vi "Import_labview_files.vi"(5 "Convert":bool, 6 "Role ID Array":T3[](array[typedef]), 9 "Hardware ID Array":T2[](array[typedef]), 11 "Folder of Labview files to import:":path=path "\\\\ccldas1.colorado.edu\\Data/Raw_Data/2012_06_16_Lightflash/Labview/run4.1") -> ()   [LabVIEW 2012]
uses:
  Private/Role ID.ctl
  Private/Hardware ID.ctl
  Private/Pelletron.ctl
  Public API/Post_Dust_Event.ctl
  Private/Estimate_source.ctl
  Private/File_location.ctl
  Public API/Signal.ctl
  <vilib>/addons/database/Auxilliary.llb/DB Tools Cursor Type.ctl
  <vilib>/Utility/file.llb/Read From Spreadsheet File (string).vi
  <vilib>/addons/database/Connection.llb/Conn Execute.vi
  <vilib>/addons/database/Recordset.llb/Rec Fetch Recordset Data (R).vi
  <vilib>/addons/database/Recordset.llb/Rec Destroy - Connection.vi
  <vilib>/addons/database/_DB Variant To Data/Database Variant To Data.xnode
  <vilib>/addons/database/NI_Database_API.lvlib
panel:
  in  "Tab Control":T1(tab)
  out "Number of Labview files to be imported:":dbl
  out "Slide":u8(slide) scale=0.0..100.0
  in  "Non-standard termination for 3rd detector?":bool
  in  "Metadata file to import:":path=path "\\\\ccldas1.colorado.edu\\Data/Raw_Data/2012_06_16_Lightflash/Labview/run4.1"
  in  "Convert Metadata":bool
  out "metadata Slide":u8(slide) scale=0.0..100.0
  out "Test":bool caption="Test Database in use:"
  out "Test 2":bool=TRUE caption="Production Database in use:"
  in  "error in (no error)":errorcluster
  out "error out":errorcluster
  in  "stop":bool
  # "CCLDAS Database Import System V2.0"
  # "ODBC Connection Status:"
  # "Error Status:"
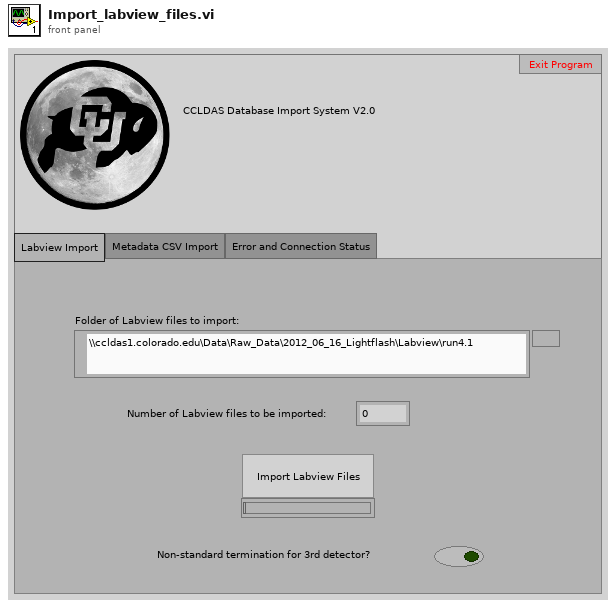
[diagram p1: front panel]
types:
  T1 = enum32{"Labview Import", "Metadata CSV Import", "Error and Connection Status"}
  T2 = typedef "Hardware ID.ctl" = enum16{"Unknown", "CSA 1", "CSA 2", "CSA 3", "CSA 4", "CSA 5", "CSA 6"}
  T3 = typedef "Role ID.ctl" = enum16{"First_Detector", "Second_Detector", "Third_Detector", "LeCroy_CH1", "LeCroy_CH2", "LeCroy_CH3", "LeCroy_CH4", "PSU"}
  T4 = typedef "Post_Dust_Event.ctl" = cluster{"Dust Event ID":i64, "Integer Timestamp":i64, "Velocity":sgl, "Mass":sgl, "Charge":sgl, "Radius":sgl, "Passed_3rd_Detector":i8, "Experiment Settings":dbl, "Pelletron ID":i32, "Estimate Source":T5, "Estimate Quality":sgl, "File Location":T6, "id_dust_info":dbl}
  T5 = typedef "Estimate_source.ctl" = i8
  T6 = typedef "File_location.ctl" = i8
  T7 = typedef "Signal.ctl" = cluster{"Signal ID":i64, "Time Stamp":timestamp, "Dust Event ID":i64, "Role ID":T3, "Data":sgl[], "Signal Length":i32, "dt":sgl, "Offset":dbl, "Hardware ID":T2}
  T8 = typedef "Pelletron.ctl" = cluster{"ID":i32, "Integer Timestamp":u64, "High Voltage":sgl, "+ High Voltage Supply":sgl, "- High Voltage Supply":sgl, "HV Control Difference":sgl, "Vacuum Pressure":sgl, "Radiation":sgl, "Column Current":sgl, "Lost Charge":sgl, "Chain Current":sgl, "Control High Voltage":sgl}
  T9 = typedef "NI_Database_API.lvlib/DB Tools Cursor Type.ctl" = enum16{"forward-only", "keyset", "dynamic", "static"}
  T10 = typedef "dust type.ctl" = cluster{"Dust info id":dbl, "Integer Timestamp":i64, "Dust Type:":u16, "Dust Source Builder:":u16, "Notes:":string, "Date of last dust soruce change:":timestamp, "Initial Dust Mass:":dbl, "Final Dust Mass:":dbl}
  T11 = typedef "NI_Database_API.lvlib/Conn ObjectReference.ctl" = refnum<k1>
  T12 = typedef "NI_Database_API.lvlib/Rec ObjectReference.ctl" = refnum<k1>
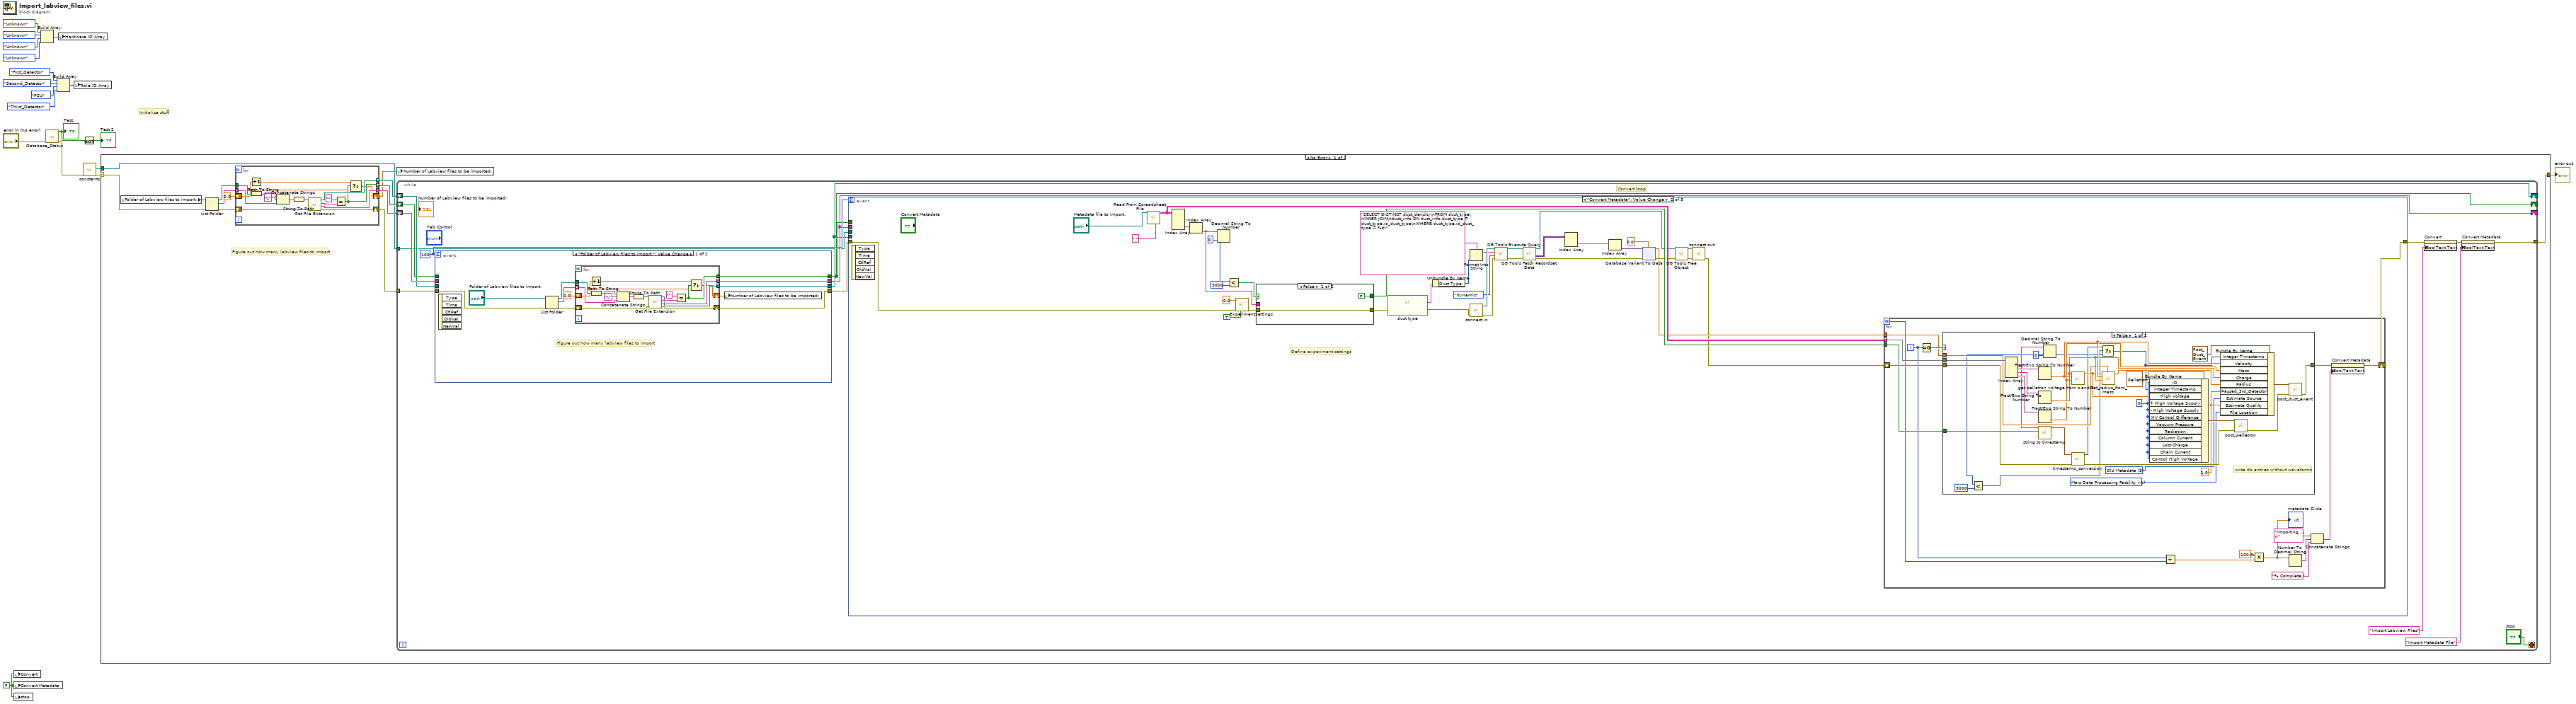
[diagram p0: block diagram]
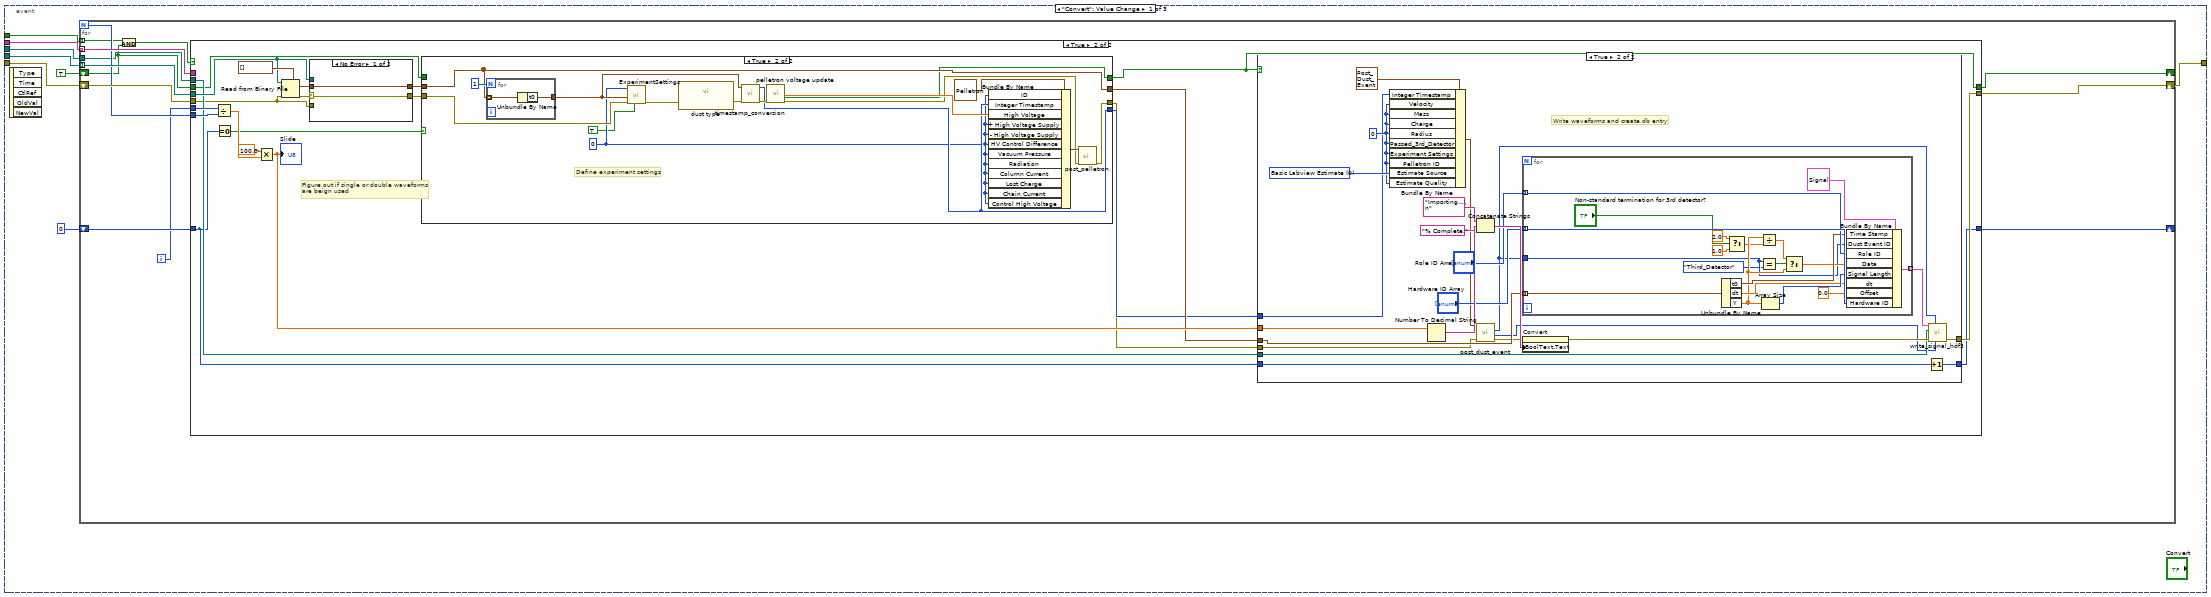
[diagram p2: hidden frame]
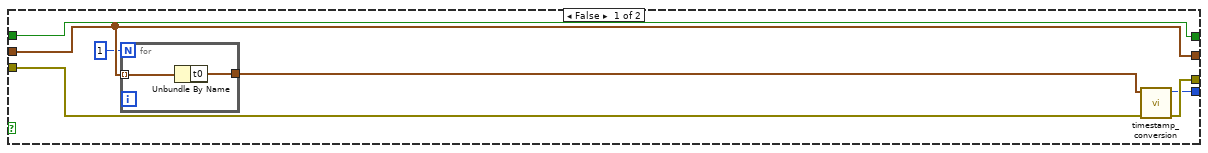
[diagram p5: hidden frame]
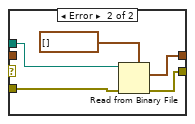
[diagram p6: hidden frame]
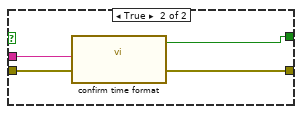
[diagram p7: hidden frame]
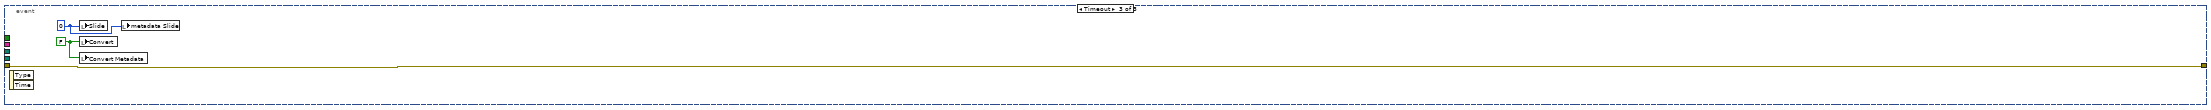
[diagram p9: hidden frame]
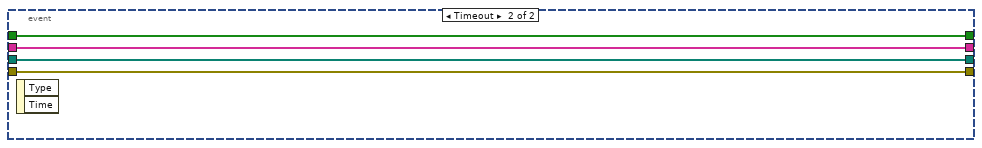
[diagram p10: hidden frame]
diagram:
  w1 = FALSE ("Convert")
  # "Initialize stuff"
  n1 = local write "Convert"(w1) -> ()
  n2 = local write "Convert Metadata"(w1) -> ()
  n3 = local write "stop"(w1) -> ()
  n4 = Build Array(Hardware_ID."Unknown" ("Hardware ID 1"), Hardware_ID."Unknown" ("Hardware ID 2"), Hardware_ID."Unknown" ("Hardware ID 3"), Hardware_ID."Unknown" ("Hardware ID 4")) -> (w12:T2[])
  n5 = call "Database_Status.vi"("error in (no error)"="error in (no error)") -> ("error out"=w3:errorcluster, "Test Database"=w5:bool)  [unwired: 9 in]
  "Test" <- w5
  n6 = Build Array(Role_ID."First_Detector" ("Role ID 1"), Role_ID."Second_Detector" ("Role ID 2"), Role_ID."PSU" ("Role ID 4"), Role_ID."Third_Detector" ("Role ID 3")) -> (w11:T3[])
  n7 = local write "Hardware ID Array"(w12) -> ()
  n8 = local write "Role ID Array"(w11) -> ()
  n9 = Not(x=w5) -> (.not. x?=→"Test 2":bool)
  n10 = call "constants.vi"("error in (no error)"=w3) -> ("error out"=w10:errorcluster, "file path for Signal .hdf5 files"=w7:path)  [unwired: 4 in, 5 out]
  n11 = case shown="No Error" w10 {
    selector: w10 -> [w19 w345]
    tunnel: [w31 w345] -> w2
    tunnel: w7 -> [w20 _]
    frame No Error {
      # "Figure out how many labview files to import"
      n12 = local read "Folder of Labview files to import:"() -> (w26:path)
      n13 = List Folder(path=w26, error in=w19) -> (path out=w29:path, filenames=w30:string[], error out=w28:errorcluster)  [unwired: 2 in, 1 out]
      n14 = for {
        tunnel: w30 -> [w42] mode=indexing
        tunnel: w29 -> [w41]
        tunnel: [w39] -> w23 mode=indexing
        shift-right: [w37] -> w25
        shift-left: w28 -> [w38]
        tunnel: [w36] -> w22 mode=indexing
        tunnel: [w35] -> w24 mode=indexing
        shift-right: [w33] -> w21
        shift-left: 0.0 -> [w32]
        n15 = Increment(x=w32) -> (x+1=w34:dbl)
        n16 = Path To String(path=w41) -> (string=w44:string)
        n17 = Concatenate Strings(w44, "\\" ("x"), w42) -> (w45:string)
        n18 = String To Path(string=w45) -> (path=w40:path)
        n19 = call <vilib>:"Get File Extension.vi"("error in (no error)"=w38, "file"=w40) -> ("error out"=w37:errorcluster, "filename without extension"=w36:string, "lowercase file extension"=w46:string, "dup file"=w39:path)  [unwired: 6 in]
        n20 = Equal?(x="" ("lowercase file extension"), y=w46) -> (x = y?=w35:bool)
        n21 = Select(t=w34, s=w35, f=w32) -> (s? t:f=w33:dbl)
      }
      n22 = local write "Number of Labview files to be imported:"(w21) -> ()
      n23 = while {
        tunnel: [w49] -> w31
        tunnel: w25 -> [w63]
        shift-right: [w59] -> _
        shift-left: w23 -> [w55]
        shift-right: [w58] -> _
        shift-left: w24 -> [w54]
        shift-right: [w57] -> _
        shift-left: w22 -> [w56]
        tunnel: w20 -> [w51]
        stop <- "stop" stop-if-true
        w61 = 100
        # "Convert loop"
        n24 = event shown="[0] \"Folder of Labview files to import:\": Value Change" {
          selector: _ -> [_ _]
          dyn-events: _ -> [_ _]
          timeout: w61 -> [_ _]
          tunnel: w63 -> [w324 w344]
          tunnel: [w320 w342] -> w59
          tunnel: [w318 w344] -> w62
          tunnel: [w317 w343] -> w57
          tunnel: [w316 w341] -> w58
          tunnel: w56 -> [_ w343]
          tunnel: w55 -> [_ w342]
          tunnel: w54 -> [_ w341]
          event "Folder of Labview files to import:": Value Change {
            # "Figure out how many labview files to import"
            n25 = event-data() -> ()  [unwired: 1 in, 5 out]
            n26 = List Folder(path="Folder of Labview files to import:", error in=w324) -> (path out=w321:path, filenames=w322:string[], error out=w319:errorcluster)  [unwired: 2 in, 1 out]
            n27 = for {
              tunnel: w322 -> [w335] mode=indexing
              tunnel: w321 -> [w334]
              tunnel: [w332] -> w320 mode=indexing
              shift-right: [w330] -> w318
              shift-left: w319 -> [w331]
              tunnel: [w329] -> w317 mode=indexing
              tunnel: [w328] -> w316 mode=indexing
              shift-right: [w326] -> w314
              shift-left: 0.0 -> [w325]
              n28 = Increment(x=w325) -> (x+1=w327:dbl)
              n29 = Path To String(path=w334) -> (string=w337:string)
              n30 = Concatenate Strings(w337, "\\" ("x"), w335) -> (w338:string)
              n31 = String To Path(string=w338) -> (path=w333:path)
              n32 = call <vilib>:"Get File Extension.vi"("error in (no error)"=w331, "file"=w333) -> ("error out"=w330:errorcluster, "filename without extension"=w329:string, "lowercase file extension"=w339:string, "dup file"=w332:path)  [unwired: 6 in]
              n33 = Equal?(x="" ("lowercase file extension"), y=w339) -> (x = y?=w328:bool)
              n34 = Select(t=w327, s=w328, f=w325) -> (s? t:f=w326:dbl)
            }
            n35 = local write "Number of Labview files to be imported:"(w314) -> ()
          }
          event Timeout {
            n36 = event-data() -> ()  [unwired: 1 in, 2 out]
          }
        }
        n37 = event shown="[1] \"Convert Metadata\": Value Change" {
          selector: _ -> [_ _ _]
          dyn-events: _ -> [_ _ _]
          timeout: w61 -> [_ _ _]
          tunnel: [w71 w196 w313] -> w53
          tunnel: w59 -> [w70 _ _]
          tunnel: w62 -> [w69 w221 w313]
          tunnel: w57 -> [w68 _ _]
          tunnel: w58 -> [w67 _ _]
          tunnel: w51 -> [w65 _ _]
          event "Convert": Value Change {
            n38 = event-data() -> ()  [unwired: 1 in, 5 out]
            n39 = for {
              N -> [w78]
              shift-right: [w84] -> w71
              shift-left: w69 -> [w81]
              tunnel: w70 -> [w83] mode=indexing
              tunnel: w68 -> [w82] mode=indexing
              tunnel: w67 -> [w73] mode=indexing
              shift-right: [w79] -> _
              shift-left: 0 ("Offset") -> [w80]
              tunnel: w65 -> [w77]
              shift-right: [w75] -> _
              shift-left: TRUE ("OK") -> [w74]
              i -> [w76]
              n40 = And(x=w73, y=w74) -> (x .and. y?=w72:bool)
              n41 = case shown="True" w72 {
                tunnel: [w87 w109] -> w84
                tunnel: w83 -> [_ w100]
                tunnel: w82 -> [_ _]
                tunnel: w81 -> [w87 w95]
                tunnel: w80 -> [w86 w97]
                tunnel: [w86 w108] -> w79
                tunnel: w76 -> [_ w107]
                tunnel: w78 -> [_ w103]
                tunnel: w77 -> [_ w98]
                tunnel: [w85 w88] -> w75
                tunnel: w74 -> [w85 w90]
                frame False {
                }
                frame True {
                  # "Figure out if single or double waveforms \nare beign used"
                  n42 = Divide(x=w107, y=w103) -> (x/y=w106:dbl)
                  n43 = Equal To 0?(x=w97) -> (x = 0?=w96:bool)
                  n44 = Multiply(x=100.0, y=w106) -> (x*y=w104:dbl)
                  "Slide" <- w104
                  n45 = Read from Binary File(5:waveform(sgl)[] [], 8:w95, 11:w100) -> (0:w101:errorcluster, 2:w99:waveform(sgl)[])  [unwired: 3 in, 2 out]
                  n46 = case shown="No Error" w101 {
                    selector: w101 -> [w182 _]
                    tunnel: [w182 w186] -> w94
                    tunnel: w100 -> [_ w185]
                    tunnel: [w181 w184] -> w93
                    tunnel: w99 -> [w181 _]
                    tunnel: w95 -> [_ w183]
                    frame No Error {
                    }
                    frame Error {
                      n47 = Read from Binary File(5:waveform(dbl)[] [], 8:w183, 11:w185) -> (0:w186:errorcluster, 2:w184:waveform(dbl)[])  [unwired: 3 in, 2 out]
                    }
                  }
                  n48 = case shown="True" w96 {
                    tunnel: w94 -> [w157 w176]
                    tunnel: [w156 w169] -> w89
                    tunnel: w93 -> [w160 w173]
                    tunnel: [w160 w173] -> w92
                    tunnel: [w155 w168] -> w91
                    tunnel: [w154 w166] -> w88
                    tunnel: w90 -> [w154 _]
                    frame False {
                      n49 = for {
                        N: 1 -> [_]
                        tunnel: w160 -> [w162] mode=indexing
                        tunnel: [w161] -> w158
                        n50 = Unbundle By Name(w162) -> ("t0"=w161:timestamp)
                      }
                      n51 = call "timestamp_conversion.vi"("error in (no error)"=w157, "Time Stamp"=w158) -> ("error out"=w156:errorcluster, "Integer Time"=w155:i64)  [unwired: 7 in]
                    }
                    frame True {
                      w167 = 0 ("ID")
                      # "Define experiment settings"
                      n52 = for {
                        N: 1 -> [_]
                        tunnel: w173 -> [w180] mode=indexing
                        tunnel: [w179] -> w174
                        n53 = Unbundle By Name(w180) -> ("t0"=w179:timestamp)
                      }
                      n54 = call "ExperimentSettings.vi"("Enable"=TRUE, "error in (no error)"=w176, "current time"=w174, "Default Group ID"=w167) -> ("error out"=w164:errorcluster)  [unwired: 6 in, 1 out]
                      n55 = call "dust type.vi"("error in (no error)"=w164) -> ("error out"=w163:errorcluster)  [unwired: 15 in, 3 out]
                      n56 = call "timestamp_conversion.vi"("error in (no error)"=w163, "Time Stamp"=w174) -> ("error out"=w171:errorcluster, "Integer Time"=w168:i64)  [unwired: 7 in]
                      n57 = call "pelletron voltage update.vi"("error in (no error)"=w171) -> ("Pelletron Voltage"=w172:dbl, "Continue"=w166:bool, "error out"=w170:errorcluster)  [unwired: 15 in, 1 out]
                      n58 = Bundle By Name(cluster=T8 {"ID"=8, "Integer Timestamp"=2, "High Voltage"=3.0, "+ High Voltage Supply"=4.0, "- High Voltage Supply"=5.0, "HV Control Difference"=6.0, "Vacuum Pressure"=7.0, "Radiation"=8.0, "Column Current"=9.0, "Lost Charge"=54.0, "Chain Current"=3.0, "Control High Voltage"=0.0} ("Pelletron Data"), "ID"=w167, "Integer Timestamp"=w168, "High Voltage"=w172, "+ High Voltage Supply"=w167, "- High Voltage Supply"=w167, "HV Control Difference"=w167, "Vacuum Pressure"=w167, "Radiation"=w167, "Column Current"=w167, "Lost Charge"=w167, "Chain Current"=w167, "Control High Voltage"=w167) -> (w177:T8)
                      n59 = call "post_pelletron.vi"("error in (no error)"=w170, "Pelletron Data"=w177) -> ("error out"=w169:errorcluster)  [unwired: 8 in, 1 out]
                    }
                  }
                  n60 = case shown="True" w88 {
                    tunnel: [w111 w134] -> w109
                    tunnel: [w110 w132] -> w108
                    tunnel: w104 -> [_ w126]
                    tunnel: w98 -> [_ w123]
                    tunnel: w97 -> [_ w114]
                    tunnel: w92 -> [_ w122]
                    tunnel: w91 -> [w110 w116]
                    tunnel: w89 -> [w111 w112]
                    frame False {
                    }
                    frame True {
                      w118 = 0
                      w119 = T5 0 items=["Basic Labview Estimate", "IDL Estimate From Andrew", "IDL Estimate From Keith", ""] ("Estimate Source")
                      # "Write waveforms and create db entry"
                      n61 = Bundle By Name(cluster=T4 {"Dust Event ID"=0, "Integer Timestamp"=0, "Velocity"=0.0, "Mass"=0.0, "Charge"=0.0, "Radius"=0.0, "Passed_3rd_Detector"=0, "Experiment Settings"=0.0, "Pelletron ID"=0, "Estimate Source"=0, "Estimate Quality"=0.0, "File Location"=0, "id_dust_info"=0.0} ("Cluster"), "Integer Timestamp"=w116, "Velocity"=w118, "Mass"=w118, "Charge"=w118, "Radius"=w118, "Passed_3rd_Detector"=w118, "Experiment Settings"=w118, "Pelletron ID"=w118, "Estimate Source"=w119, "Estimate Quality"=w118) -> (w117:T4)
                      n62 = Number To Decimal String(number=w126) -> (decimal integer string=w130:string)  [unwired: 1 in]
                      n63 = Concatenate Strings("Importing...\n" ("string"), w130, "% Complete." ("string")) -> (w127:string)
                      n64 = call "post_dust_event.vi"("error in (no error)"=w112, "Cluster"=w117) -> ("error out"=w121:errorcluster, "Experiment Settings"=w115:i32, "Dust Event ID"=w113:i32)  [unwired: 6 in, 1 out]
                      n65 = for {
                        tunnel: w122 -> [w145] mode=indexing
                        tunnel: "Role ID Array" -> [w150] mode=indexing
                        tunnel: "Hardware ID Array" -> [w151] mode=indexing
                        tunnel: [w152] -> w133 mode=indexing
                        tunnel: w113 -> [w140]
                        n66 = Unbundle By Name(w145) -> ("t0"=w147:timestamp, "dt"=w148:dbl, "Y"=w142:dbl[])
                        n67 = Select(t=2.0, s="Non-standard termination for 3rd detector?", f=1.0) -> (s? t:f=w138:dbl)
                        n68 = Divide(x=w142, y=w138) -> (x/y=w143:dbl[])
                        n69 = Equal?(x=w140, y=Role_ID."Third_Detector" ("Role ID 4")) -> (x = y?=w141:bool)
                        n70 = Array Size(array=w142) -> (size(s)=w149:i32)
                        n71 = Select(t=w143, s=w141, f=w142) -> (s? t:f=w144:dbl[])
                        n72 = Bundle By Name(cluster=T7 {"Signal ID"=0, "Time Stamp"=timestamp(0 s since 1904-01-01), "Dust Event ID"=0, "Role ID"=enum."First_Detector", "Data"=[], "Signal Length"=0, "dt"=0.0, "Offset"=0.0, "Hardware ID"=enum."Unknown"} ("Signal"), "Time Stamp"=w147, "Dust Event ID"=w140, "Role ID"=w150, "Data"=w144, "Signal Length"=w149, "dt"=w148, "Offset"=0.0, "Hardware ID"=w151) -> (w152:T7)
                      }
                      n73 = property on="Convert" class="Bool (strict)"(error in=w121, "BoolText.Text"=w127) -> (error out=w131:errorcluster)  [unwired: 1 in, 1 out]
                      n74 = Increment(x=w114) -> (x+1=w132:i64)
                      n75 = call "write_signal_hdf5.vi"("Experiment Settings ID"=w115, "Index"=w113, "error in"=w131, "Save Path"=w123, "Signal array"=w133) -> ("error out"=w134:errorcluster)  [unwired: 5 in, 1 out]
                    }
                  }
                }
              }
            }
          }
          event "Convert Metadata": Value Change {
            # "Define experiment settings"
            n76 = event-data() -> ()  [unwired: 1 in, 5 out]
            n77 = call-poly <vilib>:"Read From Spreadsheet File.vi"("delimiter (\\t)"="," ("delimiter (\\t)"), "file path (dialog if empty)"="Metadata file to import:") -> ("all rows"=w216:string[][])  [unwired: 5 in, 4 out]
            n78 = Index Array(array=w216) -> (element #2=w219:string[])  [unwired: 4 in, 1 out]
            n79 = Index Array(array=w219) -> (element=w191:string)  [unwired: 1 in]
            n80 = Decimal String To Number(string=w191, default (0L)=i64 0 ("default (0 I32)")) -> (number=w189:i64)  [unwired: 1 in, 1 out]
            n81 = Less?(x=w189, y=i64 3000) -> (x < y?=w190:bool)
            n82 = call "ExperimentSettings.vi"("Enable"=TRUE, "error in (no error)"=w221, "Default Group ID"=sgl 0.0 ("Estimate Quality")) -> ("error out"=w218:errorcluster)  [unwired: 7 in, 1 out]
            n83 = case shown="False" w190 {
              tunnel: w191 -> [_ w230]
              tunnel: w218 -> [w226 w229]
              tunnel: [w226 w228] -> w217
              tunnel: [FALSE ("Use UTC") w227] -> w215
              frame False {
              }
              frame True {
                n84 = call "confirm time format.vi"("String timestamp"=w230, "error in (no error)"=w229) -> ("Use UTC"=w227:bool, "error out"=w228:errorcluster)  [unwired: 16 in]
              }
            }
            n85 = call "dust type.vi"("error in (no error)"=w217) -> ("output cluster 2"=w222:T10, "error out"=w195:errorcluster)  [unwired: 15 in, 2 out]
            n86 = Unbundle By Name(w222) -> ("Dust Type:"=w203:u16)
            n87 = Format Into String(format string="SELECT DISTINCT dust_density\nFROM dust_type\nINNER JOIN\ndust_info ON dust_info.dust_type = dust_type.id_dust_type\nWHERE dust_type.id_dust_type = %d;" ("string"), w203) -> (resulting string=w202:string)  [unwired: 2 in, 1 out]
            n88 = call "connect in.vi"("error in (no error)"=w195) -> ("error out"=w208:errorcluster, "Database Connection"=w209:T11)  [unwired: 6 in, 1 out]
            n89 = call-poly <vilib>:"DB Tools Execute Query.vi"("error in (no error)"=w208, "cursor type"=DB_Tools_Cursor_Type."dynamic", "SQL query"=w202, "connection reference"=w209) -> ("error out"=w213:errorcluster, "recordset reference"=w214:T12)  [unwired: 4 in]
            n90 = call-poly <vilib>:"DB Tools Fetch Recordset Data.vi"("error in (no error)"=w213, "recordset reference"=w214) -> ("error out"=w211:errorcluster, "recordset data"=w199:variant[][], "recordset reference out"=w212:T12)  [unwired: 3 in]
            n91 = Index Array(array=w199) -> (element=w198:variant[])  [unwired: 2 in]
            n92 = Index Array(array=w198) -> (element=w201:variant)  [unwired: 1 in]
            n93 = xnode "Database Variant To Data"("database variant"=w201, "error in"=w211, "type"=0.0) -> ("data"=w197:dbl, "error out"=w210:errorcluster)
            n94 = call-poly <vilib>:"DB Tools Free Object.vi"("error in (no error)"=w210, "recordset reference"=w212) -> ("error out"=w205:errorcluster, "connection reference"=w207:T11)  [unwired: 8 in]
            n95 = call "connect out.vi"("error in (no error)"=w205, "connection reference"=w207) -> ("error out"=w194:errorcluster)  [unwired: 9 in]
            n96 = for {
              N -> [w272]
              shift-right: [w263] -> w196
              shift-left: w194 -> [w277]
              tunnel: w216 -> [w276] mode=indexing
              tunnel: w215 -> [w275]
              tunnel: w197 -> [w270]
              i -> [w271]
              n97 = Equal To 0?(x=w271) -> (x = 0?=w278:bool)
              n98 = case shown="False" w278 {
                tunnel: w277 -> [w287 w310]
                tunnel: [w296 w310] -> w264
                tunnel: w276 -> [w300 _]
                tunnel: w275 -> [w299 _]
                tunnel: w270 -> [w288 _]
                frame False {
                  w297 = sgl 1.0 ("Estimate Quality")
                  w301 = T5 3 items=["No Shot"=-1, "Basic Labview Estimate"=0, "IDL Estimate From Andrew"=1, "IDL Estimate From Keith"=2, "Old Metadata"=3] ("Estimate Source")
                  w302 = T6 -1 items=["Mars Data Processing Factility"=-1, "Local Cache "=0, "Storage"=1] ("File Location")
                  w307 = 0 ("ID")
                  # "write db entries without waveforms"
                  n99 = Index Array(array=w300) -> (element #1=w285:string, element #2=w295:string, element #3=w294:string, element #4=w293:string)  [unwired: 4 in]
                  n100 = Fract/Exp String To Number(string=w295) -> (number=w291:dbl)  [unwired: 3 in, 1 out]
                  n101 = Fract/Exp String To Number(string=w294) -> (number=w292:dbl)  [unwired: 3 in, 1 out]
                  n102 = Fract/Exp String To Number(string=w293) -> (number=w289:dbl)  [unwired: 3 in, 1 out]
                  n103 = call "string to timestamp.vi"("is UTC (F)"=w299, "string"=w285) -> ("time stamp"=w298:timestamp)  [unwired: 9 in]
                  n104 = Decimal String To Number(string=w285, default (0L)=i64 0 ("default (0 I32)")) -> (number=w280:i64)  [unwired: 1 in, 1 out]
                  n105 = Less?(x=w280, y=i64 3000) -> (x < y?=w279:bool)
                  n106 = call "get pelletron voltage from c and v.vi"("Mass"=w289, "Velocity"=w291, "Charge"=w292) -> ("High Voltage (MV)"=w290:sgl)  [unwired: 8 in]
                  n107 = call "timestamp_conversion.vi"("error in (no error)"=w287, "Time Stamp"=w298) -> ("error out"=w306:errorcluster, "Integer Time"=w284:i64)  [unwired: 7 in]
                  n108 = Select(t=w284, s=w279, f=w280) -> (s? t:f=w283:i64)
                  n109 = call "Get_radius_from_mass.vi"("Density"=w288, "Charge"=w292, "Velocity"=w291, "High Voltage (MV)"=w290) -> ("Radius"=w286:dbl)  [unwired: 6 in, 1 out]
                  n110 = Bundle By Name(cluster=T8 {"ID"=8, "Integer Timestamp"=2, "High Voltage"=3.0, "+ High Voltage Supply"=4.0, "- High Voltage Supply"=5.0, "HV Control Difference"=6.0, "Vacuum Pressure"=7.0, "Radiation"=8.0, "Column Current"=9.0, "Lost Charge"=54.0, "Chain Current"=3.0, "Control High Voltage"=0.0} ("Pelletron Data"), "ID"=w307, "Integer Timestamp"=w283, "High Voltage"=w290, "+ High Voltage Supply"=w307, "- High Voltage Supply"=w307, "HV Control Difference"=w307, "Vacuum Pressure"=w307, "Radiation"=w307, "Column Current"=w307, "Lost Charge"=w307, "Chain Current"=w307, "Control High Voltage"=w307) -> (w308:T8)
                  n111 = Bundle By Name(cluster=T4 {"Dust Event ID"=0, "Integer Timestamp"=0, "Velocity"=0.0, "Mass"=0.0, "Charge"=0.0, "Radius"=0.0, "Passed_3rd_Detector"=0, "Experiment Settings"=0.0, "Pelletron ID"=0, "Estimate Source"=0, "Estimate Quality"=0.0, "File Location"=0, "id_dust_info"=0.0} ("Cluster"), "Integer Timestamp"=w283, "Velocity"=w291, "Mass"=w289, "Charge"=w292, "Radius"=w286, "Passed_3rd_Detector"=w297, "Estimate Source"=w301, "Estimate Quality"=w297, "File Location"=w302) -> (w304:T4)
                  n112 = call "post_pelletron.vi"("error in (no error)"=w306, "Pelletron Data"=w308) -> ("error out"=w305:errorcluster)  [unwired: 8 in, 1 out]
                  n113 = call "post_dust_event.vi"("error in (no error)"=w305, "Cluster"=w304) -> ("error out"=w296:errorcluster)  [unwired: 6 in, 3 out]
                }
                frame True {
                }
              }
              n114 = Divide(x=w271, y=w272) -> (x/y=w274:dbl)
              n115 = Multiply(x=100.0, y=w274) -> (x*y=w267:dbl)
              "metadata Slide" <- w267
              n116 = Number To Decimal String(number=w267) -> (decimal integer string=w269:string)  [unwired: 1 in]
              n117 = Concatenate Strings("Importing...\n" ("string"), w269, "% Complete." ("string")) -> (w265:string)
              n118 = property on="Convert Metadata" class="Bool (strict)"(error in=w264, "BoolText.Text"=w265) -> (error out=w263:errorcluster)  [unwired: 1 in, 1 out]
            }
          }
          event Timeout {
            w312 = u8 0 ("Slide")
            w311 = FALSE ("Convert")
            n119 = event-data() -> ()  [unwired: 1 in, 2 out]
            n120 = local write "Slide"(w312) -> ()
            n121 = local write "Convert"(w311) -> ()
            n122 = local write "Convert Metadata"(w311) -> ()
            n123 = local write "metadata Slide"(w312) -> ()
          }
        }
        n124 = property on="Convert" class="Bool (strict)"(error in=w53, "BoolText.Text"="Import Labview Files" ("Boolean Text.Text")) -> (error out=w50:errorcluster)  [unwired: 1 in, 1 out]
        n125 = property on="Convert Metadata" class="Bool (strict)"(error in=w50, "BoolText.Text"="Import Metadata File" ("Boolean Text.Text")) -> (error out=w49:errorcluster)  [unwired: 1 in, 1 out]
      }
    }
    frame Error {
    }
  }
  "error out" <- w2
